vi "FrontPanel.vi"() -> ()   [LabVIEW 2017, in "AODControl.lvlib"]
uses:
  AODControl.lvlib
  LoadControl.ctl
  InterfaceReferences.ctl
  ExitButton.ctl
  AODSettings.ctl
  AODPointDefinition.ctl
  ListOfPoints.ctl
  <vilib>/Utility/error.llb/DialogType.ctl
  DecodifyFrequency(Array).vi
  MessageQueue/QueueOperations/Enqueue Message (Array).vi
  AODGlobals.vi
  MessageQueue/QueueOperations/Enqueue Message (Single).vi
  MovePoint.vi
  AddPoint.vi
  RemovePoint.vi
  ReplaceList.vi
  AddPoints.vi
  <vilib>/Utility/file.llb/Write To Spreadsheet File (DBL).vi
  <vilib>/Utility/file.llb/Read From Spreadsheet File (DBL).vi
  CodifyFrequency(Array).vi
  MessageQueue/MessageQueue.lvlib
panel:
  in  "Reset Sequence":bool
  out "Sequence":dbl[][][](array[numeric])
  in  "Frame":i32 max=10 step=1
  out "Frames":i32 step=1
  in  "SaveFrame":bool
  in  "Play":bool
  in  "Playing Time":dbl step=0.1
  in  "Tasks":T1={"XTask"="Frequency1", "YTask"="Frequency2"}
  out "Dynamic":bool
  in  "Speed Y":dbl
  in  "Speed Scale":dbl step=0.1
  in  "Speed X":dbl
  in  "Speed Rotate":dbl step=0.1
  in  "Rotate":bool
  in  "Exit Button":T2
  in  "?":T3
  in  "Save List":bool
  in  "Load List":T4
  in  "New List":dbl[][](array[numeric])
  in  "ReplaceList":bool
  out "Number Of Points":i32
  out "Points":dbl[][](array[numeric])
  in  "Add":bool
  out "Display":cluster{dbl[], dbl[]}(graph)
  in  "Move":bool
  in  "Index":i32 min=0 max=1
  in  "Remove":bool
  in  "Y":dbl
  in  "X":dbl
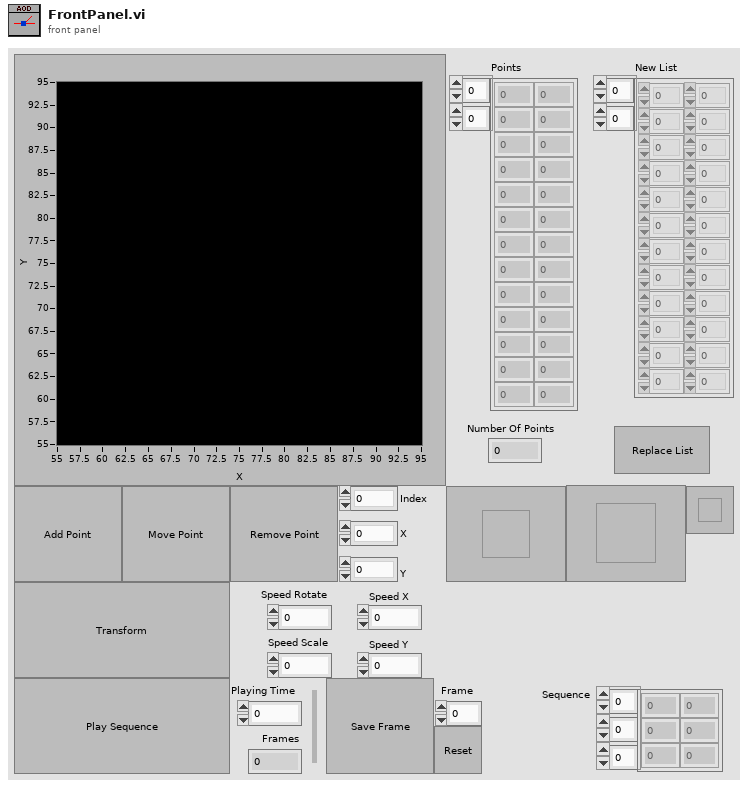
[diagram p1: front panel]
types:
  T1 = typedef "AODControl.lvlib/AODSettings.ctl" = cluster{"XTask":refnum<k21>, "YTask":refnum<k21>}
  T2 = typedef "AODControl.lvlib/ExitButton.ctl" = bool
  T3 = typedef "AODControl.lvlib/InterfaceReferences.ctl" = cluster{"AOD Points Display":refnum<vi>, "AOD Array":refnum<vi>, "AOD Array Size":refnum<vi>, "Replace Array List":refnum<vi>, "Replace List":refnum<vi>, "Remove":refnum<vi>, "Index":refnum<vi>, "Move":refnum<vi>, "X":refnum<vi>, "Y":refnum<vi>, "Add":refnum<vi>, "Load":refnum<vi>, "Save":refnum<vi>, "Exit":refnum<vi>, "Dynamic":refnum<vi>, "Rotate":refnum<vi>, "Rotation Speed":refnum<vi>, "Scaling Speed":refnum<vi>, "X Trans Speed":refnum<vi>, "Y Trans Speed":refnum<vi>, "Movie Array":refnum<vi>}
  T4 = typedef "AODControl.lvlib/LoadControl.ctl" = bool
  T5 = typedef "AODControl.lvlib/ListOfPoints.ctl" = cluster{"X":u32[], "Y":u32[], "Amp":dbl[]}
  T6 = typedef "AODControl.lvlib/AODPointDefinition.ctl" = cluster{"Freq X":dbl, "Freq Y":dbl, "Index":i32, "Ampitude":dbl}
  T7 = typedef "AODControl.lvlib/MessageQueue.lvlib/All Message Queues.ctl" = cluster{" AOD Interface":refnum<queue>}
  T8 = typedef "DialogType.ctl" = u16
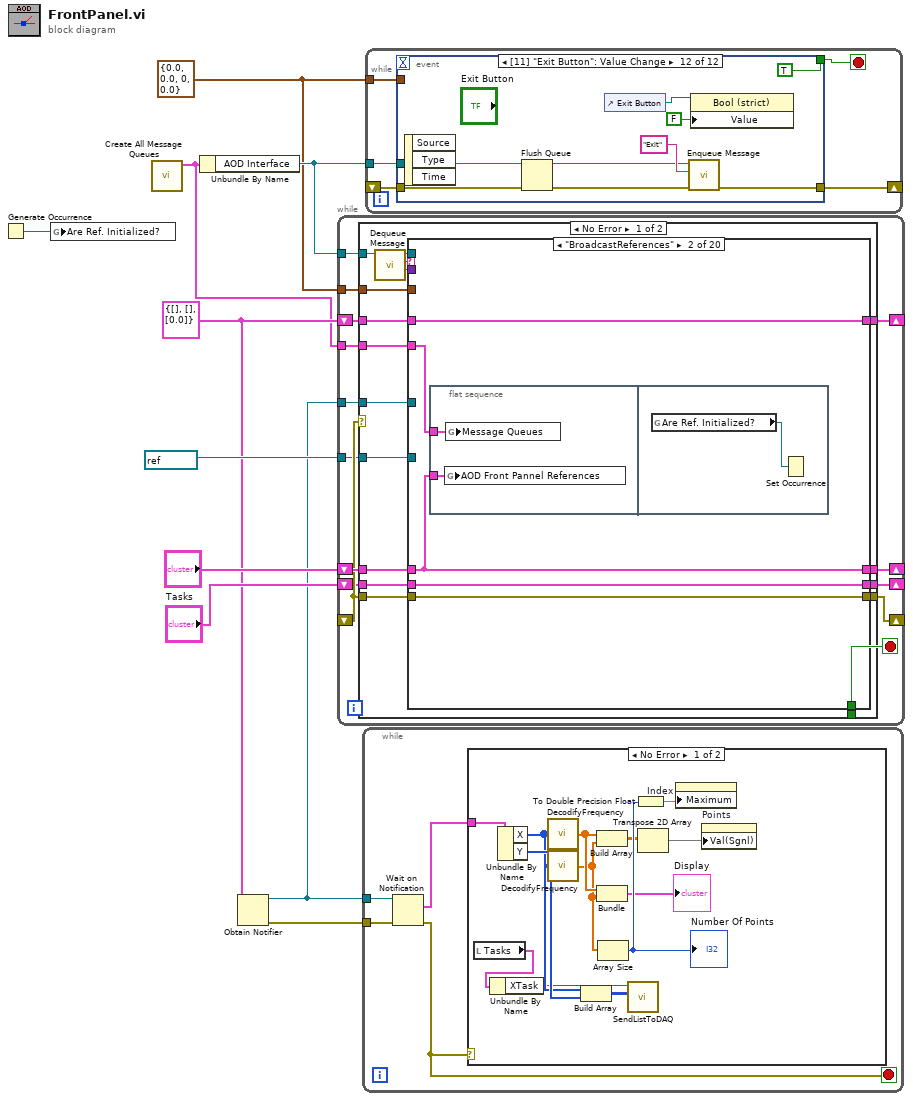
[diagram p0: block diagram]
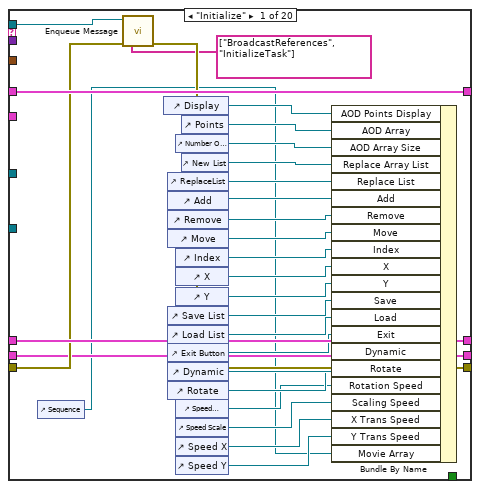
[diagram p3: hidden frame]
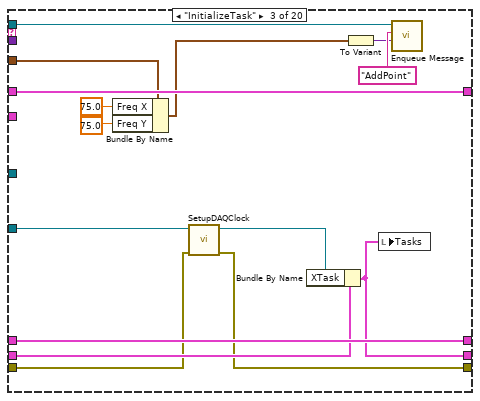
[diagram p4: hidden frame]
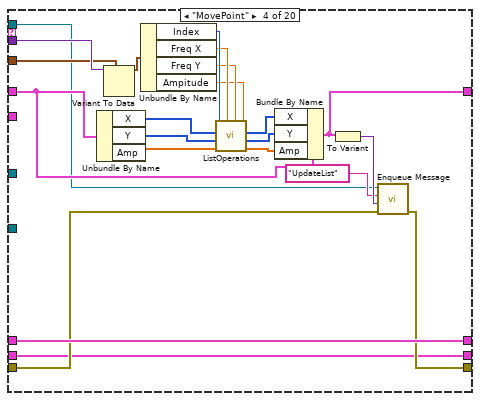
[diagram p5: hidden frame]
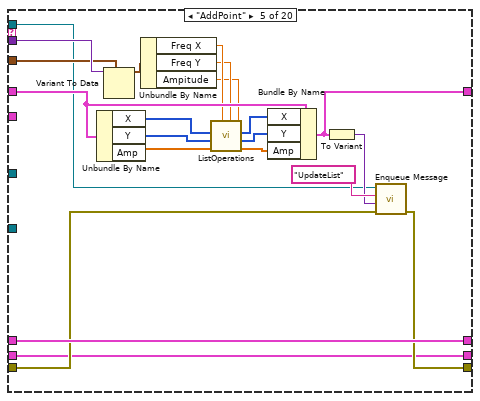
[diagram p6: hidden frame]
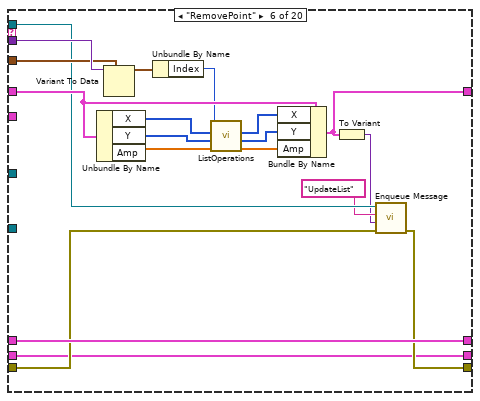
[diagram p7: hidden frame]
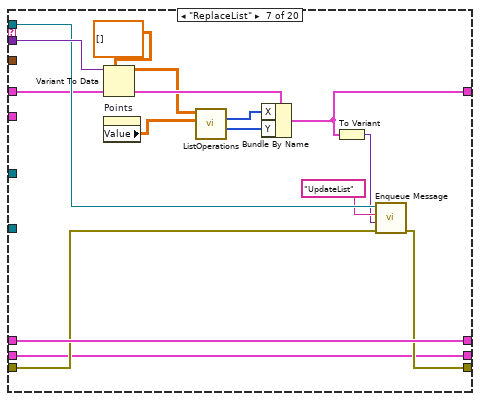
[diagram p8: hidden frame]
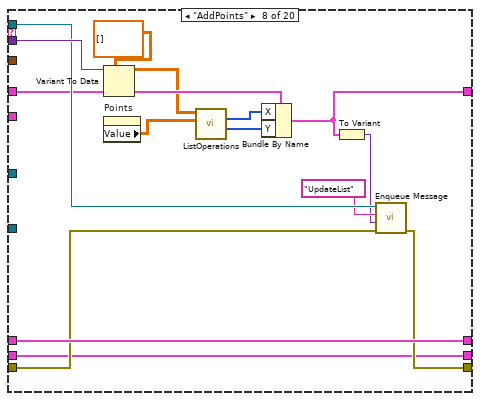
[diagram p9: hidden frame]
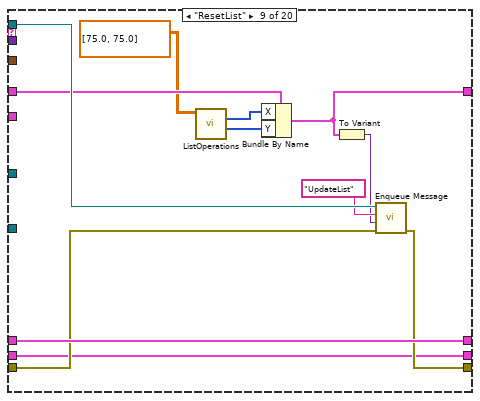
[diagram p10: hidden frame]
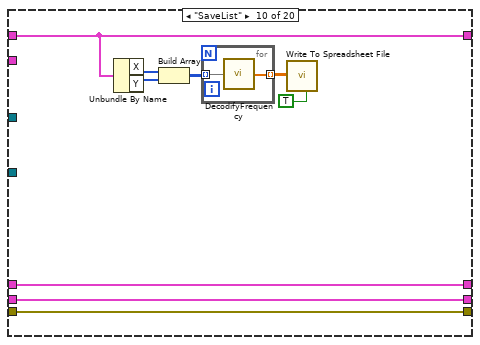
[diagram p11: hidden frame]
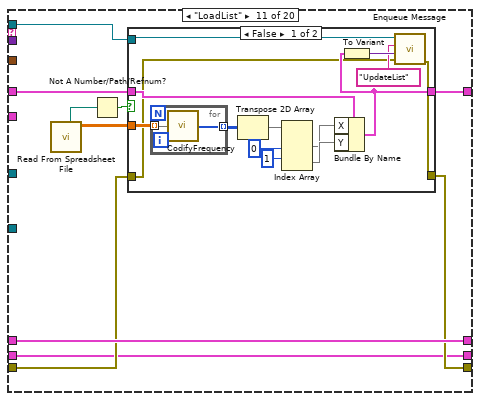
[diagram p12: hidden frame]
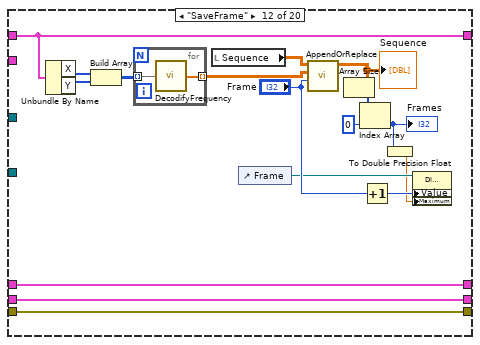
[diagram p14: hidden frame]
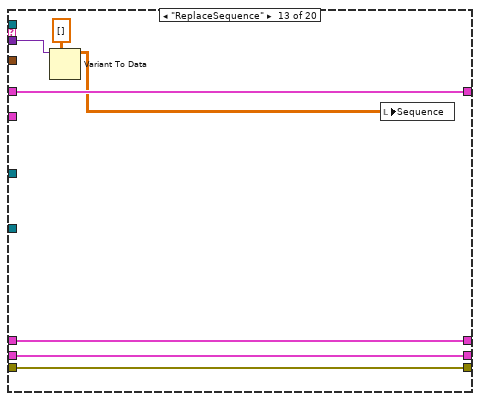
[diagram p15: hidden frame]
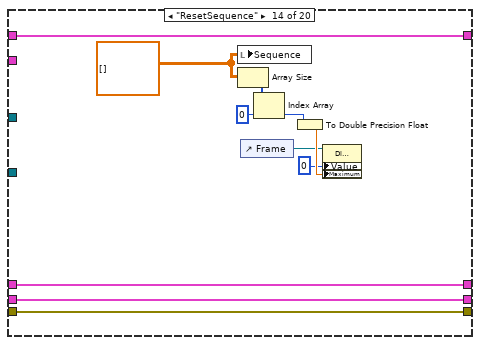
[diagram p16: hidden frame]
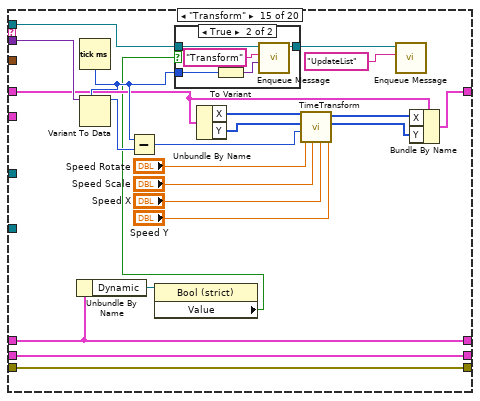
[diagram p17: hidden frame]
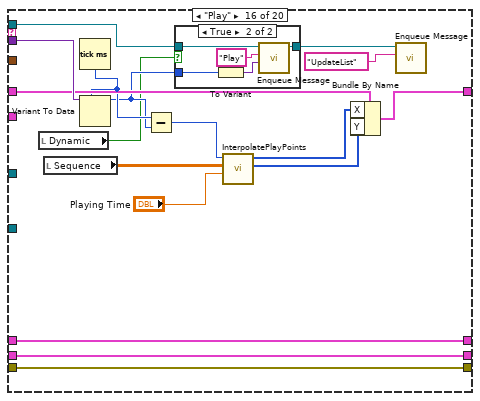
[diagram p19: hidden frame]
diagram:
  w5 = T5 {"X"=[], "Y"=[], "Amp"=[0.0]} ("Cluster")
  w9 = T6 {"Freq X"=0.0, "Freq Y"=0.0, "Index"=0, "Ampitude"=0.0}
  n1 = Generate Occurrence() -> (w1:refnum<k4>)
  n2 = global write "AODGlobals.vi" "Are Ref. Initialized?"(w1) -> ()
  n3 = call "Create All Message Queues.vi"() -> ("Message Queues out"=w2:T7)  [unwired: 10 in, 1 out]
  n4 = Unbundle By Name(w2) -> ("AOD Interface"=w10:refnum<queue>)
  n5 = Obtain Notifier(notification data type=w5) -> (notifier out=w3:refnum<notifier>, error out=w4:errorcluster)  [unwired: 2 in, 2 out]
  n6 = while {
    tunnel: w10 -> [w13]
    shift-right: [w23] -> _
    shift-left: w5 -> [w24]
    tunnel: w9 -> [w21]
    shift-right: [w19] -> _
    shift-left: "?" -> [w20]
    shift-right: [w18] -> _
    shift-left: _ -> [w17]
    shift-right: [w15] -> _
    shift-left: "Tasks" -> [w16]
    tunnel: refnum<k21> "AOD" ("task/channels in") -> [w14]
    tunnel: w3 -> [w12]
    tunnel: w2 -> [w11]
    stop <- w22 stop-if-true
    n7 = case shown="No Error" w17 {
      tunnel: w13 -> [w30 _]
      tunnel: w24 -> [w41 w349]
      tunnel: [w40 w349] -> w23
      tunnel: [w39 _] -> w22
      tunnel: w21 -> [w38 _]
      tunnel: w20 -> [w37 w350]
      tunnel: [w36 w350] -> w19
      tunnel: [w35 w351] -> w18
      tunnel: w17 -> [w34 w352]
      tunnel: w16 -> [w31 w348]
      tunnel: [w33 w348] -> w15
      tunnel: w14 -> [w32 _]
      tunnel: w12 -> [w26 _]
      tunnel: w11 -> [w25 _]
      frame No Error {
        n8 = call "Dequeue Message.vi"("Message Queue"=w30) -> ("Message Data"=w28:variant, "Message"=w27:string, "dup Message Queue"=w29:refnum<queue>)  [unwired: 7 in, 1 out]
        n9 = case shown="\"BroadcastReferences\"" w27 {
          tunnel: w29 -> [w58 _ w84 w98 w120 w144 w169 w184 w197 _ w217 _ _ _ w293 w316 _ _ _ _]
          tunnel: w28 -> [_ _ _ w115 w136 w155 w170 w185 _ _ _ _ w257 _ w292 w315 _ _ _ _]
          tunnel: w41 -> [w57 w75 w93 w112 w133 w152 w163 w178 w192 w205 w215 w250 w262 w273 w287 w307 w327 w335 w343 w347]
          tunnel: [w57 w75 w93 w99 w121 w142 w162 w177 w191 w205 w214 w250 w262 w273 w286 w306 w327 w335 w343 w347] -> w40
          tunnel: [_ _ _ _ _ _ _ _ _ _ _ _ _ _ _ _ _ _ TRUE _] -> w39
          tunnel: w38 -> [_ _ w83 w114 w135 w154 _ _ _ _ _ _ _ _ _ _ _ _ _ _]
          tunnel: w37 -> [w70 w73 w92 w97 w119 w140 w160 w175 w190 w206 w218 w248 w261 w272 w276 w312 w330 w334 w341 w346]
          tunnel: [w54 w73 w92 w97 w119 w140 w160 w175 w190 w206 w218 w248 w261 w272 w276 w312 w330 w334 w341 w346] -> w36
          tunnel: [w52 w72 w87 w95 w117 w138 w158 w173 w188 w199 w212 w246 w259 w270 w294 w317 w325 w333 w337 w345] -> w35
          tunnel: w34 -> [w53 w72 w88 w96 w118 w139 w159 w174 w189 w199 w213 w246 w259 w270 w294 w317 w326 w333 w338 w345]
          tunnel: [w51 w74 w79 w94 w116 w137 w157 w172 w187 w198 w209 w247 w260 w271 w295 w318 w329 w332 w340 w344] -> w33
          tunnel: w32 -> [_ _ w91 _ _ _ _ _ _ _ _ _ _ _ _ _ _ _ _ _]
          tunnel: w31 -> [w51 w74 w90 w94 w116 w137 w157 w172 w187 w198 w209 w247 w260 w271 w295 w318 w329 w332 w340 w344]
          tunnel: w26 -> [_ _ _ _ _ _ _ _ _ _ _ _ _ _ _ _ w328 _ w336 _]
          tunnel: w25 -> [_ w71 _ _ _ _ _ _ _ _ _ _ _ _ _ _ _ _ _ _]
          frame "Initialize" {
            n10 = control-ref of="Sequence"() -> (w42:refnum<vi>)
            n11 = call-poly "Enqueue Message.vi"("error in (no error)"=w53, "Message Array"=string[] ["BroadcastReferences", "InitializeTask"], "Message Queue"=w58) -> ("error out"=w52:errorcluster)  [unwired: 7 in, 1 out]
            n12 = control-ref of="Display"() -> (w69:refnum<vi>)
            n13 = control-ref of="ReplaceList"() -> (w65:refnum<vi>)
            n14 = control-ref of="Add"() -> (w64:refnum<vi>)
            n15 = control-ref of="Remove"() -> (w63:refnum<vi>)
            n16 = control-ref of="Move"() -> (w62:refnum<vi>)
            n17 = control-ref of="Save List"() -> (w56:refnum<vi>)
            n18 = control-ref of="Load List"() -> (w55:refnum<vi>)
            n19 = control-ref of="Exit Button"() -> (w48:refnum<vi>)
            n20 = control-ref of="Dynamic"() -> (w49:refnum<vi>)
            n21 = control-ref of="Rotate"() -> (w47:refnum<vi>)
            n22 = control-ref of="Number Of Points"() -> (w67:refnum<vi>)
            n23 = control-ref of="Index"() -> (w61:refnum<vi>)
            n24 = control-ref of="X"() -> (w60:refnum<vi>)
            n25 = control-ref of="Y"() -> (w59:refnum<vi>)
            n26 = control-ref of="Speed Rotate"() -> (w46:refnum<vi>)
            n27 = control-ref of="Speed Scale"() -> (w45:refnum<vi>)
            n28 = control-ref of="Speed X"() -> (w44:refnum<vi>)
            n29 = control-ref of="Speed Y"() -> (w43:refnum<vi>)
            n30 = control-ref of="Points"() -> (w68:refnum<vi>)
            n31 = control-ref of="New List"() -> (w66:refnum<vi>)
            n32 = Bundle By Name(cluster=w70, "AOD Points Display"=w69, "AOD Array"=w68, "AOD Array Size"=w67, "Replace Array List"=w66, "Replace List"=w65, "Add"=w64, "Remove"=w63, "Move"=w62, "Index"=w61, "X"=w60, "Y"=w59, "Save"=w56, "Load"=w55, "Exit"=w48, "Dynamic"=w49, "Rotate"=w47, "Rotation Speed"=w46, "Scaling Speed"=w45, "X Trans Speed"=w44, "Y Trans Speed"=w43, "Movie Array"=w42) -> (w54:T3)
          }
          frame "BroadcastReferences" {
            n33 = flat-sequence {
              tunnel: w73 -> [w77]
              tunnel: w71 -> [w76]
              frame #0 {
                n34 = global write "AODGlobals.vi" "AOD Front Pannel References"(w77) -> ()
                n35 = global write "AODGlobals.vi" "Message Queues"(w76) -> ()
              }
              frame #1 {
                n36 = global read "AODGlobals.vi" "Are Ref. Initialized?"() -> (w78:refnum<k4>)
                n37 = Set Occurrence(w78) -> ()
              }
            }
          }
          frame "InitializeTask" {
            n38 = Bundle By Name(cluster=w83, "Freq X"=75.0, "Freq Y"=75.0 ("Freq X")) -> (w80:T6)
            n39 = call "SetupDAQClock.vi"("error in"=w88, "task/channels in"=w91) -> ("error out"=w87:errorcluster, "task out"=w89:refnum<k21>)  [unwired: 8 in]
            n40 = Bundle By Name(cluster=w90, "XTask"=w89) -> (w79:T1)
            n41 = To Variant(anything=w80) -> (Variant=w85:variant)
            n42 = local write "Tasks"(w79) -> ()
            n43 = call-poly "Enqueue Message.vi"("Message Data"=w85, "Message"="AddPoint", "Message Queue"=w84) -> ()  [unwired: 7 in, 2 out]
          }
          frame "MovePoint" {
            n44 = Unbundle By Name(w112) -> ("X"=w107:u32[], "Y"=w106:u32[], "Amp"=w105:dbl[])
            n45 = Variant To Data(type=w114, Variant=w115) -> (data=w113:T6)  [unwired: 1 in, 1 out]
            n46 = Unbundle By Name(w113) -> ("Index"=w111:i32, "Freq X"=w110:dbl, "Freq Y"=w109:dbl, "Ampitude"=w108:dbl)
            n47 = call-poly "ListOperations.vi"("Ampitude"=w108, "Freq Y"=w109, "Freq X"=w110, "Amp in"=w105, "Y in"=w106, "X in"=w107, "Index"=w111) -> ("Amp out"=w103:dbl[], "Y out"=w102:u32[], "X out"=w104:u32[])  [unwired: 2 in]
            n48 = Bundle By Name(cluster=w112, "X"=w104, "Y"=w102, "Amp"=w103) -> (w99:T5)
            n49 = To Variant(anything=w99) -> (Variant=w101:variant)
            n50 = call-poly "Enqueue Message.vi"("error in (no error)"=w96, "Message Data"=w101, "Message"="UpdateList", "Message Queue"=w98) -> ("error out"=w95:errorcluster)  [unwired: 6 in, 1 out]
          }
          frame "AddPoint" {
            n51 = Unbundle By Name(w133) -> ("X"=w129:u32[], "Y"=w128:u32[], "Amp"=w127:dbl[])
            n52 = Variant To Data(type=w135, Variant=w136) -> (data=w134:T6)  [unwired: 1 in, 1 out]
            n53 = Unbundle By Name(w134) -> ("Freq X"=w132:dbl, "Freq Y"=w131:dbl, "Ampitude"=w130:dbl)
            n54 = call-poly "ListOperations.vi"("Ampitude"=w130, "Freq Y"=w131, "Freq X"=w132, "Amp in"=w127, "Y in"=w128, "X in"=w129) -> ("Amp out"=w124:dbl[], "Y out"=w125:u32[], "X out"=w126:u32[])  [unwired: 3 in]
            n55 = Bundle By Name(cluster=w133, "X"=w126, "Y"=w125, "Amp"=w124) -> (w121:T5)
            n56 = To Variant(anything=w121) -> (Variant=w122:variant)
            n57 = call-poly "Enqueue Message.vi"("error in (no error)"=w118, "Message Data"=w122, "Message"="UpdateList", "Message Queue"=w120) -> ("error out"=w117:errorcluster)  [unwired: 6 in, 1 out]
          }
          frame "RemovePoint" {
            n58 = Unbundle By Name(w152) -> ("X"=w151:u32[], "Y"=w150:u32[], "Amp"=w149:dbl[])
            n59 = Variant To Data(type=w154, Variant=w155) -> (data=w153:T6)  [unwired: 1 in, 1 out]
            n60 = Unbundle By Name(w153) -> ("Index"=w145:i32)
            n61 = call-poly "ListOperations.vi"("Amp in"=w149, "Y in"=w150, "X in"=w151, "Index"=w145) -> ("Amp out"=w146:dbl[], "Y out"=w147:u32[], "X out"=w148:u32[])  [unwired: 5 in]
            n62 = Bundle By Name(cluster=w152, "X"=w148, "Y"=w147, "Amp"=w146) -> (w142:T5)
            n63 = To Variant(anything=w142) -> (Variant=w141:variant)
            n64 = call-poly "Enqueue Message.vi"("error in (no error)"=w139, "Message Data"=w141, "Message"="UpdateList", "Message Queue"=w144) -> ("error out"=w138:errorcluster)  [unwired: 6 in, 1 out]
          }
          frame "ReplaceList" {
            n65 = Variant To Data(type=dbl[][] [] ("New List"), Variant=w170) -> (data=w161:dbl[][])  [unwired: 1 in, 1 out]
            n66 = property on="Points" class="Arr (strict)"() -> ("Value"=w156:dbl[][])  [unwired: 2 in, 2 out]
            n67 = call-poly "ListOperations.vi"("Old List"=w156, "New List"=w161) -> ("Y"=w164:u32[], "X"=w165:u32[])  [unwired: 8 in]
            n68 = Bundle By Name(cluster=w163, "X"=w165, "Y"=w164) -> (w162:T5)
            n69 = To Variant(anything=w162) -> (Variant=w167:variant)
            n70 = call-poly "Enqueue Message.vi"("error in (no error)"=w159, "Message Data"=w167, "Message"="UpdateList", "Message Queue"=w169) -> ("error out"=w158:errorcluster)  [unwired: 6 in, 1 out]
          }
          frame "AddPoints" {
            n71 = Variant To Data(type=dbl[][] [] ("New List"), Variant=w185) -> (data=w176:dbl[][])  [unwired: 1 in, 1 out]
            n72 = property on="Points" class="Arr (strict)"() -> ("Value"=w171:dbl[][])  [unwired: 2 in, 2 out]
            n73 = call-poly "ListOperations.vi"("Old List"=w171, "New List"=w176) -> ("Y"=w179:u32[], "X"=w180:u32[])  [unwired: 8 in]
            n74 = Bundle By Name(cluster=w178, "X"=w180, "Y"=w179) -> (w177:T5)
            n75 = To Variant(anything=w177) -> (Variant=w182:variant)
            n76 = call-poly "Enqueue Message.vi"("error in (no error)"=w174, "Message Data"=w182, "Message"="UpdateList", "Message Queue"=w184) -> ("error out"=w173:errorcluster)  [unwired: 6 in, 1 out]
          }
          frame "ResetList" {
            n77 = call-poly "ListOperations.vi"("New List"=dbl[][] [[75.0, 75.0]]) -> ("Y"=w193:u32[], "X"=w194:u32[])  [unwired: 9 in]
            n78 = Bundle By Name(cluster=w192, "X"=w194, "Y"=w193) -> (w191:T5)
            n79 = To Variant(anything=w191) -> (Variant=w195:variant)
            n80 = call-poly "Enqueue Message.vi"("error in (no error)"=w189, "Message Data"=w195, "Message"="UpdateList", "Message Queue"=w197) -> ("error out"=w188:errorcluster)  [unwired: 6 in, 1 out]
          }
          frame "SaveList" {
            n81 = Unbundle By Name(w205) -> ("X"=w204:u32[], "Y"=w203:u32[])
            n82 = Build Array(w204, w203) -> (w201:u32[][])
            n83 = for {
              tunnel: w201 -> [w208] mode=indexing
              tunnel: [w207] -> w202 mode=indexing
              n84 = call-poly "DecodifyFrequency.vi"("Array 2"=w208) -> ("Array"=w207:dbl[])
            }
            n85 = call-poly <vilib>:"Write To Spreadsheet File.vi"("transpose? (no:F)"=TRUE, "2D data"=w202) -> ()  [unwired: 6 in, 1 out]
          }
          frame "LoadList" {
            n86 = call-poly <vilib>:"Read From Spreadsheet File.vi"() -> ("all rows"=w216:dbl[][], "new file path (Not A Path if cancelled)"=w211:path)  [unwired: 7 in, 3 out]
            n87 = Not A Number/Path/Refnum?(number/path/refnum=w211) -> (NaN/Path/Refnum?=w210:bool)
            n88 = case shown="False" w210 {
              tunnel: w217 -> [w232 _]
              tunnel: w216 -> [w229 _]
              tunnel: w215 -> [w224 w235]
              tunnel: [w221 w235] -> w214
              tunnel: w213 -> [w220 w236]
              tunnel: [w219 w236] -> w212
              frame False {
                n89 = for {
                  tunnel: w229 -> [w234] mode=indexing
                  tunnel: [w233] -> w228 mode=indexing
                  n90 = call-poly "CodifyFrequency.vi"("Array"=w234) -> ("Array 2"=w233:u32[])
                }
                n91 = Transpose 2D Array(2D array=w228) -> (transposed array=w227:u32[][])
                n92 = Index Array(array=w227, index (row) #1=0 ("index (row)"), index (row) #2=1 ("index (row)")) -> (element #1=w222:u32[], element #2=w223:u32[])  [unwired: 2 in]
                n93 = Bundle By Name(cluster=w224, "X"=w222, "Y"=w223) -> (w221:T5)
                n94 = To Variant(anything=w221) -> (Variant=w231:variant)
                n95 = call-poly "Enqueue Message.vi"("error in (no error)"=w220, "Message Data"=w231, "Message"="UpdateList", "Message Queue"=w232) -> ("error out"=w219:errorcluster)  [unwired: 6 in, 1 out]
              }
              frame True {
              }
            }
          }
          frame "SaveFrame" {
            n96 = Unbundle By Name(w250) -> ("X"=w251:u32[], "Y"=w252:u32[])
            n97 = Build Array(w251, w252) -> (w253:u32[][])
            n98 = for {
              tunnel: w253 -> [w255] mode=indexing
              tunnel: [w254] -> w244 mode=indexing
              n99 = call-poly "DecodifyFrequency.vi"("Array 2"=w255) -> ("Array"=w254:dbl[])
            }
            n100 = local read "Sequence"() -> (w245:dbl[][][])
            n101 = control-ref of="Frame"() -> (w240:refnum<vi>)
            n102 = call "AppendOrReplace.vi"("index 2"="Frame", "new element/subarray 2"=w244, "Sequence 2"=w245) -> ("Sequence"=w243:dbl[][][])  [unwired: 8 in]
            "Sequence" <- w243
            n103 = Array Size(array=w243) -> (size(s)=w249:i32[])
            n104 = Index Array(array=w249, index=0) -> (element=w238:i32)
            "Frames" <- w238
            n105 = Increment(x="Frame") -> (x+1=w239:i32)
            n106 = To Double Precision Float(number=w238) -> (double precision float=w237:dbl)
            n107 = property class="DigNum (strict)"(reference=w240, "Value"=w239, "Maximum"=w237) -> ()  [unwired: 1 in, 2 out]
          }
          frame "ReplaceSequence" {
            n108 = Variant To Data(type=dbl[][][] [] ("Sequence"), Variant=w257) -> (data=w256:dbl[][][])  [unwired: 1 in, 1 out]
            n109 = local write "Sequence"(w256) -> ()
          }
          frame "ResetSequence" {
            w263 = dbl[][][] [] ("Sequence")
            n110 = local write "Sequence"(w263) -> ()
            n111 = Array Size(array=w263) -> (size(s)=w266:i32[])
            n112 = control-ref of="Frame"() -> (w264:refnum<vi>)
            n113 = Index Array(array=w266, index=0) -> (element=w268:i32)
            n114 = To Double Precision Float(number=w268) -> (double precision float=w269:dbl)
            n115 = property class="DigNum (strict)"(reference=w264, "Value"=0 ("Frame"), "Maximum"=w269) -> ()  [unwired: 1 in, 2 out]
          }
          frame "Transform" {
            n116 = Unbundle By Name(w276) -> ("Dynamic"=w275:refnum<vi>)
            n117 = Tick Count (ms)() -> (millisecond timer value=w291:u32)
            n118 = Variant To Data(type=w291, Variant=w292) -> (data=w290:u32)  [unwired: 1 in, 1 out]
            n119 = Subtract(x=w291, y=w290) -> (x-y=w277:u32)
            n120 = property class="Bool (strict)"(reference=w275) -> ("Value"=w274:bool)  [unwired: 1 in, 2 out]
            n121 = case shown="True" w274 {
              tunnel: w293 -> [w296 w301]
              tunnel: w291 -> [_ w298]
              tunnel: [w296 w297] -> w289
              frame False {
              }
              frame True {
                n122 = To Variant(anything=w298) -> (Variant=w299:variant)
                n123 = call-poly "Enqueue Message.vi"("Message Data"=w299, "Message"="Transform", "Message Queue"=w301) -> ("dup Message Queue"=w297:refnum<queue>)  [unwired: 7 in, 1 out]
              }
            }
            n124 = Unbundle By Name(w287) -> ("X"=w285:u32[], "Y"=w284:u32[])
            n125 = call "TimeTransform.vi"("Speed Y"="Speed Y", "Speed X"="Speed X", "Speed Scale"="Speed Scale", "Speed Rotate"="Speed Rotate", "Elapsed Time"=w277, "Y"=w284, "X"=w285) -> ("Y out"=w282:u32[], "X out"=w283:u32[])  [unwired: 3 in]
            n126 = call-poly "Enqueue Message.vi"("Message"="UpdateList", "Message Queue"=w289) -> ()  [unwired: 8 in, 2 out]
            n127 = Bundle By Name(cluster=w287, "X"=w283, "Y"=w282) -> (w286:T5)
          }
          frame "Play" {
            n128 = local read "Dynamic"() -> (w303:bool)
            n129 = local read "Sequence"() -> (w302:dbl[][][])
            n130 = Tick Count (ms)() -> (millisecond timer value=w305:u32)
            n131 = Variant To Data(type=w305, Variant=w315) -> (data=w304:u32)  [unwired: 1 in, 1 out]
            n132 = Subtract(x=w305, y=w304) -> (x-y=w311:u32)
            n133 = case shown="True" w303 {
              tunnel: w316 -> [w319 w324]
              tunnel: w304 -> [_ w321]
              tunnel: [w319 w320] -> w314
              frame False {
              }
              frame True {
                n134 = To Variant(anything=w321) -> (Variant=w322:variant)
                n135 = call-poly "Enqueue Message.vi"("Message Data"=w322, "Message"="Play", "Message Queue"=w324) -> ("dup Message Queue"=w320:refnum<queue>)  [unwired: 7 in, 1 out]
              }
            }
            n136 = call "InterpolatePlayPoints.vi"("Total Playing Time (sec)"="Playing Time", "Point List"=w302, "Ellapsed Time (ms)"=w311) -> ("Y"=w308:u32[], "X"=w309:u32[])  [unwired: 7 in]
            n137 = Bundle By Name(cluster=w307, "X"=w309, "Y"=w308) -> (w306:T5)
            n138 = call-poly "Enqueue Message.vi"("Message"="UpdateList", "Message Queue"=w314) -> ()  [unwired: 8 in, 2 out]
          }
          frame "UpdateList" {
            n139 = Send Notification(notification=w327, notifier=w328, error in (no error)=w326) -> (error out=w325:errorcluster)  [unwired: 1 out]
          }
          frame "ExitFromOutside" {
            n140 = property on="Exit Button" class="Bool (strict)"("Val(Sgnl)"=FALSE) -> ()  [unwired: 2 in, 2 out]
          }
          frame "Exit" {
            n141 = Release Notifier(notifier=w336) -> ()  [unwired: 1 in, 4 out]
            n142 = Unbundle By Name(w340) -> ("XTask"=w339:refnum<k21>)
            n143 = call "StopDAQ.vi"("error in"=w338, "Refnum in"=w339) -> ("error out"=w337:errorcluster)  [unwired: 9 in]
          }
          frame Default {
          }
        }
      }
      frame Error {
        w353 = T8 2 items=["no dialog", "OK message", "continue or stop message", "OK message + warnings", "continue/stop + warnings"] ("type of dialog (OK msg:1)")
        n144 = call <vilib>:"Simple Error Handler.vi"("type of dialog (OK msg:1)"=w353, "error in (no error)"=w352) -> ("error out"=w354:errorcluster)  [unwired: 3 in, 4 out]
        n145 = call <vilib>:"Clear Errors.vi"("error in (no error)"=w354) -> ("error out"=w351:errorcluster)  [unwired: 5 in, 1 out]
      }
    }
  }
  n146 = while {
    tunnel: w3 -> [w357]
    tunnel: w4 -> [w355]
    stop <- w358 stop-if-true
    n147 = Wait on Notification(notifier=w357, error in (no error)=w355) -> (notification=w356:T5, error out=w358:errorcluster)  [unwired: 4 out]
    n148 = case shown="No Error" w358 {
      tunnel: w356 -> [w360 _]
      frame No Error {
        n149 = local read "Tasks"() -> (w359:T1)
        n150 = Unbundle By Name(w359) -> ("XTask"=w365:refnum<k21>)
        n151 = Unbundle By Name(w360) -> ("X"=w367:u32[], "Y"=w368:u32[])
        n152 = call-poly "DecodifyFrequency.vi"("Array 2"=w367) -> ("Array"=w370:dbl[])
        n153 = call-poly "DecodifyFrequency.vi"("Array 2"=w368) -> ("Array"=w369:dbl[])
        n154 = Build Array(w367, w368) -> (w366:u32[][])
        n155 = Build Array(w370, w369) -> (w362:dbl[][])
        n156 = Bundle("Array"=w370, "Array"=w369) -> (→"Display":cluster{"Array":dbl[], "Array":dbl[]})  [unwired: 1 in]
        n157 = Array Size(array=w369) -> (size(s)=w364:i32)
        "Number Of Points" <- w364
        n158 = call "SendListToDAQ.vi"("Input"=w366, "Refnum in"=w365) -> ()  [unwired: 8 in, 2 out]
        n159 = To Double Precision Float(number=w364) -> (double precision float=w363:dbl)
        n160 = Transpose 2D Array(2D array=w362) -> (transposed array=w371:dbl[][])
        n161 = property on="Index" class="DigNum (strict)"("Maximum"=w363) -> ()  [unwired: 2 in, 2 out]
        n162 = property on="Points" class="Arr (strict)"("Val(Sgnl)"=w371) -> ()  [unwired: 2 in, 2 out]
      }
      frame Error {
      }
    }
  }
  n163 = while {
    tunnel: w10 -> [w376]
    tunnel: w9 -> [w375]
    shift-right: [w373] -> _
    shift-left: _ -> [w372]
    stop <- w374 stop-if-true
    n164 = event shown="[11] \"Exit Button\": Value Change" {
      selector: _ -> [_ _ _ _ _ _ _ _ _ _ _ _]
      dyn-events: _ -> [_ _ _ _ _ _ _ _ _ _ _ _]
      timeout: _ -> [_ _ _ _ _ _ _ _ _ _ _ _]
      tunnel: [_ _ _ _ _ _ _ _ _ _ TRUE TRUE] -> w374
      tunnel: w376 -> [w385 w395 w403 w409 w413 w417 w419 w423 w429 w434 w439 w444]
      tunnel: w375 -> [w384 w394 w402 _ _ _ _ _ _ _ _ _]
      tunnel: [w377 w386 w396 w404 w410 w414 w420 w424 _ _ w436 w447] -> w373
      tunnel: w372 -> [w378 w387 w397 w405 w411 w415 w421 w425 _ _ w437 w443]
      event "Add": Value Change {
        n165 = event-data() -> ()  [unwired: 1 in, 1 out]
        n166 = Bundle By Name(cluster=w384, "Freq X"="X", "Freq Y"="Y") -> (w383:T6)
        n167 = To Variant(anything=w383) -> (Variant=w382:variant)
        n168 = call-poly "Enqueue Message.vi"("error in (no error)"=w378, "Message Data"=w382, "Message"="AddPoint", "Message Queue"=w385) -> ("error out"=w377:errorcluster)  [unwired: 6 in, 1 out]
      }
      event "Move": Value Change {
        n169 = event-data() -> ()  [unwired: 1 in, 1 out]
        n170 = property on="X" class="DigNum (strict)"() -> ("Value"=w390:dbl)  [unwired: 2 in, 2 out]
        n171 = property on="Y" class="DigNum (strict)"() -> ("Value"=w389:dbl)  [unwired: 2 in, 2 out]
        n172 = property on="Index" class="DigNum (strict)"() -> ("Value"=w388:i32)  [unwired: 2 in, 2 out]
        n173 = Bundle By Name(cluster=w394, "Freq X"=w390, "Freq Y"=w389, "Index"=w388) -> (w393:T6)
        n174 = To Variant(anything=w393) -> (Variant=w392:variant)
        n175 = call-poly "Enqueue Message.vi"("error in (no error)"=w387, "Message Data"=w392, "Message"="MovePoint", "Message Queue"=w395) -> ("error out"=w386:errorcluster)  [unwired: 6 in, 1 out]
      }
      event "Remove": Value Change {
        n176 = event-data() -> ()  [unwired: 1 in, 1 out]
        n177 = Bundle By Name(cluster=w402, "Index"="Index") -> (w401:T6)
        n178 = To Variant(anything=w401) -> (Variant=w400:variant)
        n179 = call-poly "Enqueue Message.vi"("error in (no error)"=w397, "Message Data"=w400, "Message"="RemovePoint", "Message Queue"=w403) -> ("error out"=w396:errorcluster)  [unwired: 6 in, 1 out]
      }
      event "ReplaceList": Value Change {
        n180 = event-data() -> ()  [unwired: 1 in, 1 out]
        n181 = To Variant(anything="New List") -> (Variant=w408:variant)
        n182 = call-poly "Enqueue Message.vi"("error in (no error)"=w405, "Message Data"=w408, "Message"="ReplaceList", "Message Queue"=w409) -> ("error out"=w404:errorcluster)  [unwired: 6 in, 1 out]
      }
      event "Save List": Value Change {
        n183 = event-data() -> ()  [unwired: 1 in, 1 out]
        n184 = call-poly "Enqueue Message.vi"("error in (no error)"=w411, "Message"="SaveList", "Message Queue"=w413) -> ("error out"=w410:errorcluster)  [unwired: 7 in, 1 out]
      }
      event Value Change {
        n185 = event-data() -> ()  [unwired: 1 in, 1 out]
        n186 = call-poly "Enqueue Message.vi"("error in (no error)"=w415, "Message"="LoadList", "Message Queue"=w417) -> ("error out"=w414:errorcluster)  [unwired: 7 in, 1 out]
      }
      event "SaveFrame": Value Change {
        n187 = event-data() -> ()  [unwired: 1 in, 1 out]
        n188 = call-poly "Enqueue Message.vi"("error in (no error)"=w421, "Message"="SaveFrame", "Message Queue"=w419) -> ("error out"=w420:errorcluster)  [unwired: 7 in, 1 out]
      }
      event "Reset Sequence": Value Change {
        n189 = event-data() -> ()  [unwired: 1 in, 1 out]
        n190 = call-poly "Enqueue Message.vi"("error in (no error)"=w425, "Message"="ResetSequence", "Message Queue"=w423) -> ("error out"=w424:errorcluster)  [unwired: 7 in, 1 out]
      }
      event "Rotate": Value Change {
        n191 = event-data() -> ()  [unwired: 1 in, 1 out]
        n192 = Tick Count (ms)() -> (millisecond timer value=w426:u32)
        n193 = To Variant(anything=w426) -> (Variant=w427:variant)
        n194 = call-poly "Enqueue Message.vi"("Message Data"=w427, "Message"="Transform", "Message Queue"=w429) -> ()  [unwired: 7 in, 2 out]
        "Dynamic" <- "Rotate"
      }
      event "Play": Value Change {
        n195 = event-data() -> ()  [unwired: 1 in, 1 out]
        n196 = local write "Dynamic"("Play") -> ()
        n197 = Tick Count (ms)() -> (millisecond timer value=w432:u32)
        n198 = To Variant(anything=w432) -> (Variant=w433:variant)
        n199 = call-poly "Enqueue Message.vi"("Message Data"=w433, "Message"="Play", "Message Queue"=w434) -> ()  [unwired: 7 in, 2 out]
      }
      event Panel Close {
        n200 = event-data() -> ()  [unwired: 1 in, 1 out]
        n201 = call-poly "Enqueue Message.vi"("error in (no error)"=w437, "Message"="Exit", "Message Queue"=w439) -> ("error out"=w436:errorcluster)  [unwired: 7 in, 1 out]
      }
      event Value Change {
        n202 = event-data() -> ()  [unwired: 1 in, 3 out]
        n203 = Flush Queue(queue=w444, error in (no error)=w443) -> (queue out=w441:refnum<queue>, error out=w442:errorcluster)  [unwired: 1 out]
        n204 = control-ref of="Exit Button"() -> (w446:refnum<vi>)
        n205 = call-poly "Enqueue Message.vi"("error in (no error)"=w442, "Message"="Exit", "Message Queue"=w441) -> ("error out"=w447:errorcluster)  [unwired: 7 in, 1 out]
        n206 = property class="Bool (strict)"(reference=w446, "Value"=T2 FALSE) -> ()  [unwired: 1 in, 2 out]
      }
    }
  }
